vi "Is Concrete Class.vi"(0 "Vector Abstract Path Group in":refnum<class "Vector Abstract Path Group.lvclass">, 11 "error in (no error)":errorcluster) -> (4 "Vector Abstract Path Group out":refnum<class "Vector Abstract Path Group.lvclass">, 6 "Is Concrete Class?":bool, 15 "error out":errorcluster)   [LabVIEW 2023, in "RFFixtureCharact.Public.lvlib" / "Vector Abstract Path Group.lvclass"]
uses:
  Vector Abstract Path Group.lvclass
  Vector Abstract Path Group.lvclass/Vector Abstract Path Group.ctl
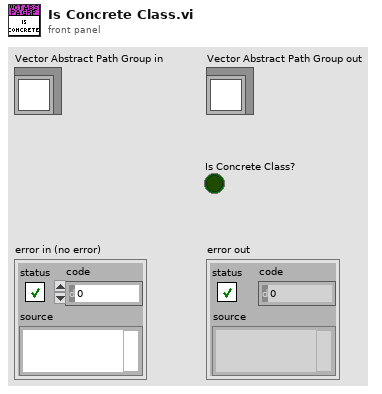
[diagram p1: front panel]
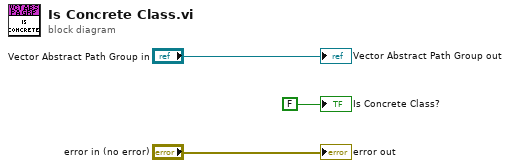
[diagram p0: block diagram]
diagram:
  "error out" <- "error in (no error)"
  "Vector Abstract Path Group out" <- "Vector Abstract Path Group in"
  "Is Concrete Class?" <- FALSE ("Is Concrete Class?")
